vi "combined2.vi"() -> ()   [LabVIEW 2020]
uses:
  C:/Users/Public/Documents/Photometrics/PMQI-LabViewSamples/Examples/2018/Dependencies/PVCamNET.dll
  Dependencies/PVCamNET.dll
panel:
  out "SavingPath":string
  out "Saving":bool
  out "Capturing":bool
  in  "seq_save":bool
  in  "seq_start":bool
  in  "Path":path
  in  "FramesToCapture":u16
  in  "Full CCD Height":u16
  in  "Full CCD Width":u16
  in  "Full CCD":bool
  in  "Get ROI":bool
  in  "Height":u16
  in  "Y":u16
  in  "Width":u16
  in  "X":u16
  out "Trigger Mode":i32
  in  "Trigger In Behaviour":string(combo)
  out "Exp. out":i32
  in  "Trigger Out Behaviour":string(combo)
  out "Boolean":bool
  in  "Scan Direction Reset":bool
  out "Scan Line Time":dbl format="%#_14g"
  in  "Scan Width":dbl
  in  "Scan Line Delay":dbl
  in  "Scan Direction":string(combo)
  in  "Scan Mode":string(combo)
  in  "Exposure Time":dbl
  in  "Live":bool
  in  "Camera Status":bool
  in  "Uninit":bool
  in  "Live stop":bool
  in  "Live start":bool
  in  "Open":bool
  # "Description:\nThis code lets the user use programmable scan\n mode for live imaging.\n\nSteps to run:\n1. Click \"Run\"\n2. Click \"Open\"\n3. Enter Exposure Time\n4. Select Scan Mode. \n5. Set Scan Line Delay or Scan Width\n6. Select Scan Direction\n7. Click \"Live start\"\n8. Click \"Live stop\"\n9. Right click on CamWindow and add a ROI.\n10. Click \"Get ROI\"\n11. Click \"Live start\"\n12. Click \"Live stop\"\n13. Right click on CamWindow and delete a ROI.\n14. Click \"Close\""
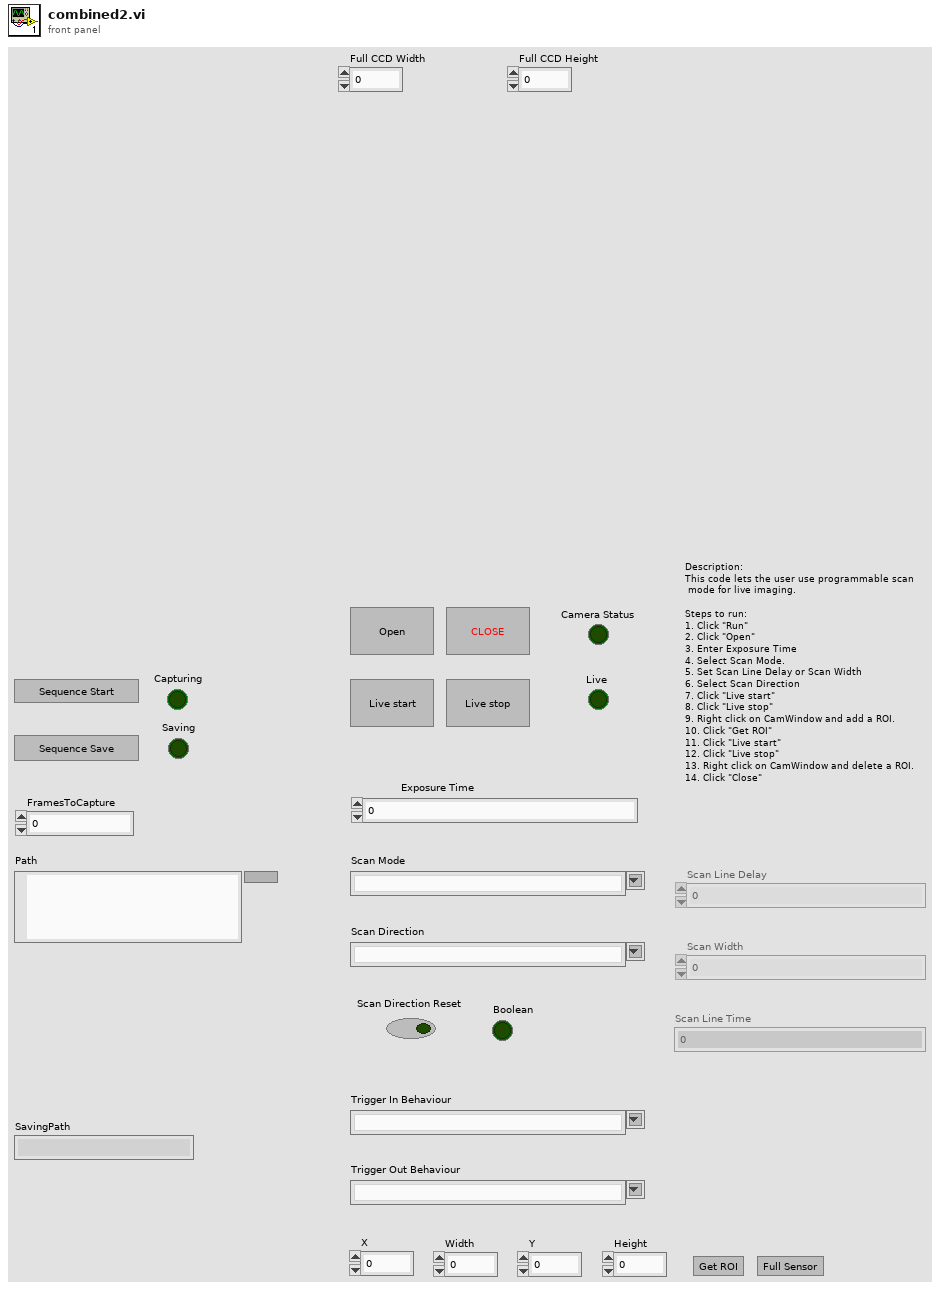
[diagram p1: front panel]
types:
  T1 = enum8{"Enabled", "Disabled", "Disabled and Grayed Out"}
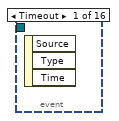
[diagram p2: hidden frame]
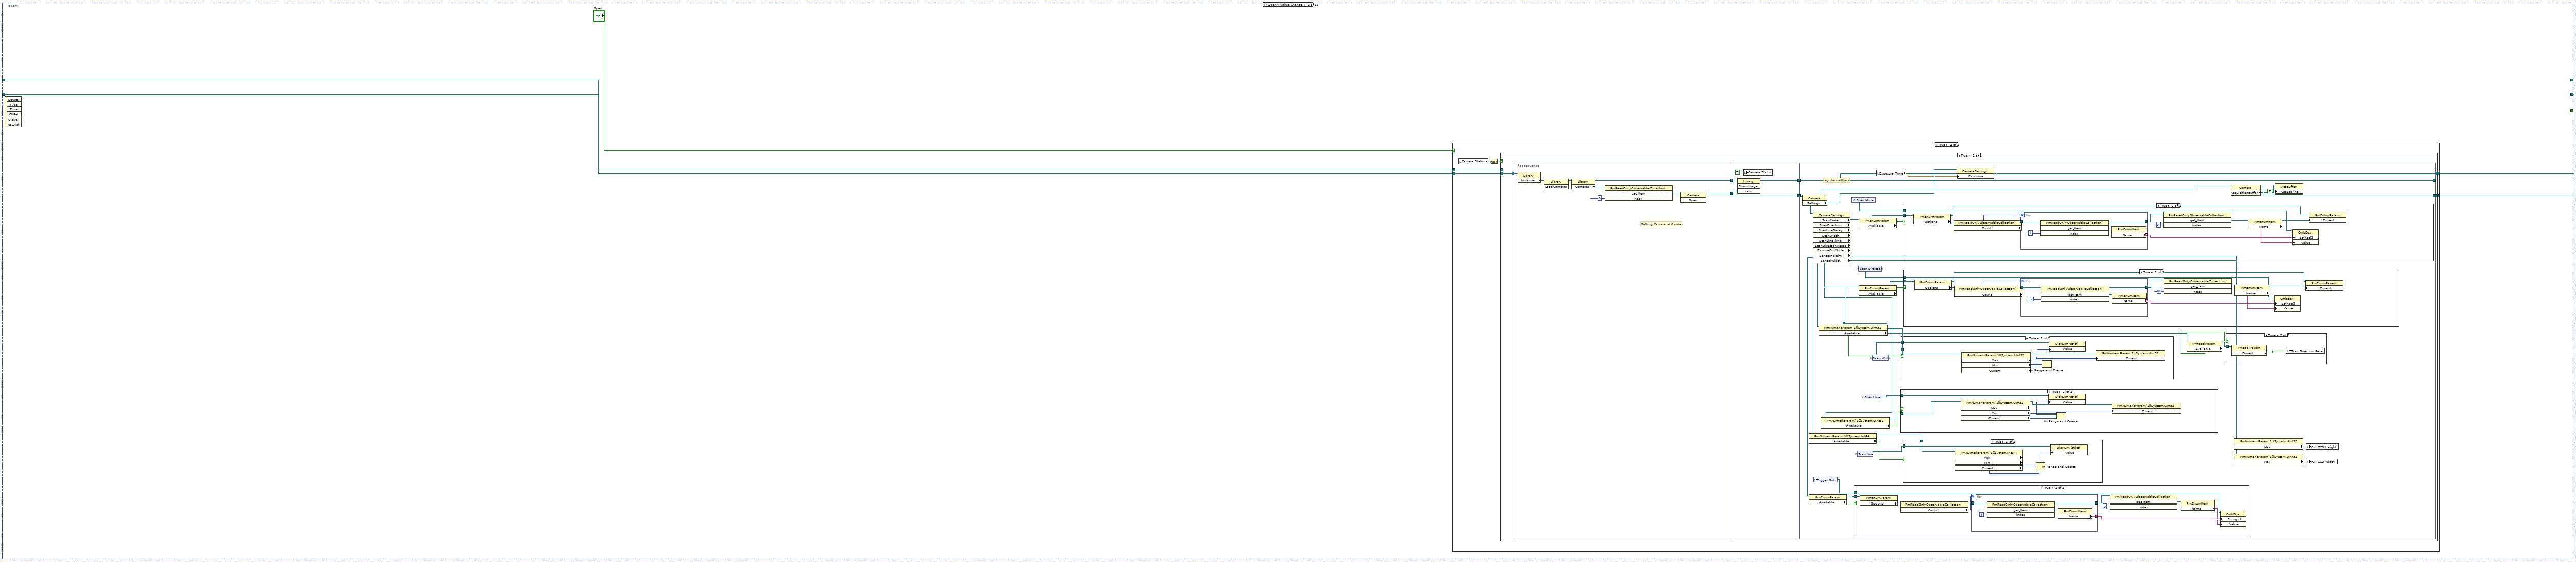
[diagram p3: hidden frame]
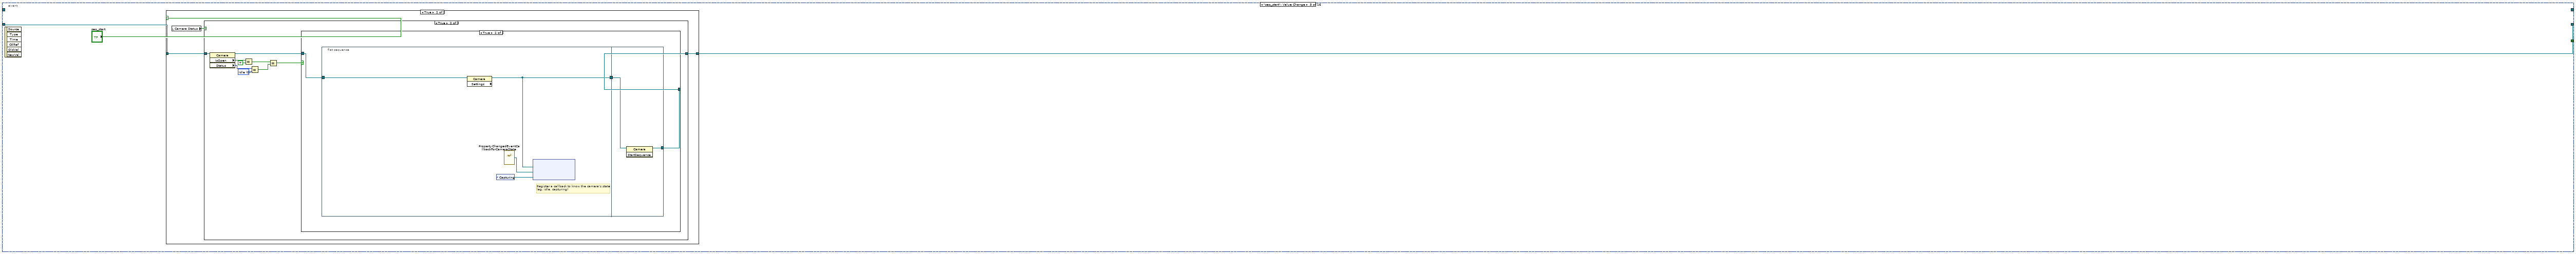
[diagram p13: hidden frame]
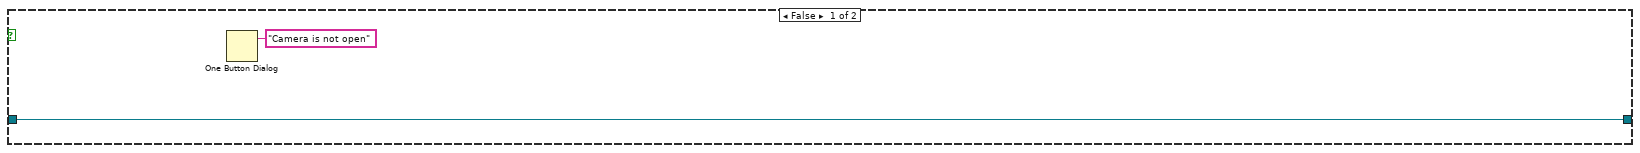
[diagram p15: hidden frame]
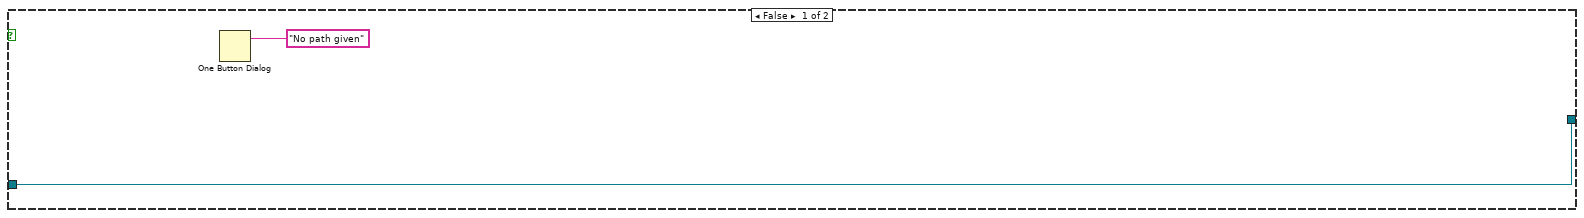
[diagram p18: hidden frame]
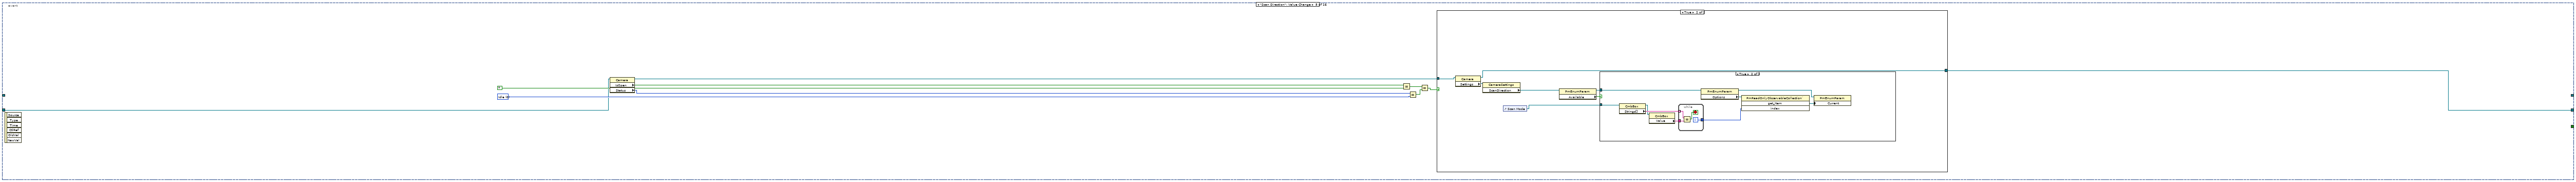
[diagram p20: hidden frame]
diagram:
  w15 = T1."Disabled and Grayed Out" ("Disabled")
  n1 = flat-sequence {
    tunnel: [w31] -> w30
    tunnel: w30 -> [w33]
    tunnel: [w32] -> w29
    tunnel: w29 -> [w859]
    frame #0 {
      n2 = property class="Library"() -> ("Instance"=w31:refnum<k24>)  [unwired: 2 in, 2 out]
    }
    frame #1 {
      n3 = while {
        tunnel: w33 -> [w38]
        shift-right: [w37] -> _
        shift-left: _ -> [w35]
        tunnel: [w36] -> w32
        stop <- w34 stop-if-true
        n4 = event shown="[3] \"seq_save\": Value Change" {
          selector: _ -> [_ _ _ _ _ _ _ _ _ _ _ _ _ _ _ _]
          dyn-events: _ -> [_ _ _ _ _ _ _ _ _ _ _ _ _ _ _ _]
          timeout: _ -> [_ _ _ _ _ _ _ _ _ _ _ _ _ _ _ _]
          tunnel: w38 -> [_ w43 _ _ _ _ _ _ w533 _ _ _ _ w776 _ w831]
          tunnel: [_ w42 w183 w214 w246 w278 w410 w474 w534 w601 w638 w711 w738 w777 w806 w832] -> w37
          tunnel: [_ w41 _ _ _ _ _ _ w533 _ _ _ _ w776 _ w831] -> w36
          tunnel: w35 -> [_ w40 w184 w213 w250 w279 w416 w476 w535 w602 w639 w712 w739 w778 w807 w833]
          tunnel: [_ _ _ _ _ _ _ _ _ _ _ _ _ _ _ w830] -> w34
          event Timeout {
            n5 = event-data() -> ()  [unwired: 1 in, 3 out]
          }
          event "Open": Value Change {
            n6 = event-data() -> ()  [unwired: 1 in, 6 out]
            n7 = case shown="True" "Open" {
              tunnel: w43 -> [w45 w51]
              tunnel: [w44 w50] -> w42
              tunnel: [w45 w49] -> w41
              tunnel: w40 -> [w44 w46]
              frame False {
              }
              frame True {
                n8 = local read "Camera Status"() -> (w48:bool)
                n9 = Not(x=w48) -> (.not. x?=w47:bool)
                n10 = case shown="True" w47 {
                  tunnel: w51 -> [w52 w58]
                  tunnel: [w53 w57] -> w50
                  tunnel: [w52 w56] -> w49
                  tunnel: w46 -> [w53 _]
                  frame False {
                  }
                  frame True {
                    n11 = flat-sequence {
                      tunnel: w58 -> [w63]
                      tunnel: [w65] -> w60
                      tunnel: [w64] -> w59
                      tunnel: w60 -> [w71]
                      tunnel: w59 -> [w72]
                      tunnel: [w72] -> w55
                      tunnel: [w70] -> w54
                      tunnel: [w111] -> w56
                      tunnel: [w91] -> w57
                      tunnel: w55 -> [w110]
                      tunnel: w54 -> [w111]
                      frame #0 {
                        # "Getting Camera at 0 index"
                        n12 = property class="Library"(reference=w63) -> ("Instance"=w62:refnum<k24>)  [unwired: 1 in, 2 out]
                        n13 = invoke class="Library" method="LoadCameras"(reference=w62) -> (reference out=w61:refnum<k24>)  [unwired: 2 in, 2 out]
                        n14 = property class="Library"(reference=w61) -> (reference out=w65:refnum<k24>, "Cameras"=w68:refnum<k24>)  [unwired: 1 in, 1 out]
                        n15 = invoke class="PmReadOnlyObservableCollection`" method="get_Item"(reference=w68, "index"=0) -> ("get_Item"=w66:refnum<k24>)  [unwired: 2 in, 3 out]
                        n16 = invoke class="Camera" method="Open"(reference=w66) -> (reference out=w64:refnum<k24>)  [unwired: 2 in, 2 out]
                      }
                      frame #1 {
                        n17 = invoke class="Library" method="ShowImage"(reference=w71, "cam"=w72) -> (reference out=w70:refnum<k24>)  [unwired: 2 in, 3 out]
                        n18 = local write "Camera Status"(TRUE ("Camera Status")) -> ()
                      }
                      frame #2 {
                        # "register callback"
                        n19 = property class="Camera"(reference=w110) -> (reference out=w92:refnum<k24>, "Settings"=w81:refnum<k24>)  [unwired: 1 in, 1 out]
                        n20 = property class="CameraSettings"(reference=w81) -> ("ScanMode"=w109:refnum<k24>, "ScanDirection"=w105:refnum<k24>, "ScanLineDelay"=w100:refnum<k24>, "ScanWidth"=w87:refnum<k24>, "ScanLineTime"=w79:refnum<k24>, "ScanDirectionReset"=w95:refnum<k24>, "ExposeOutMode"=w83:refnum<k24>, "SensorHeight"=w74:refnum<k24>, "SensorWidth"=w73:refnum<k24>)  [unwired: 1 in, 2 out]
                        n21 = property class="PmNumericParam`1[[System.Int64,"(reference=w79) -> (reference out=w77:refnum<k24>, "Available"=w78:bool)  [unwired: 1 in, 1 out]
                        n22 = property class="PmEnumParam"(reference=w83) -> (reference out=w84:refnum<k24>, "Available"=w85:bool)  [unwired: 1 in, 1 out]
                        n23 = control-ref of="Trigger Out Behaviour"() -> (w82:refnum<vi>)
                        n24 = property class="PmNumericParam`1[[System.UInt32"(reference=w100) -> (reference out=w98:refnum<k24>, "Available"=w99:bool)  [unwired: 1 in, 1 out]
                        n25 = property class="PmNumericParam`1[[System.UInt32"(reference=w87) -> (reference out=w86:refnum<k24>, "Available"=w88:bool)  [unwired: 1 in, 1 out]
                        n26 = control-ref of="Scan Mode"() -> (w106:refnum<vi>)
                        n27 = case shown="True" w85 {
                          tunnel: w84 -> [_ w121]
                          tunnel: w82 -> [_ w112]
                          frame False {
                          }
                          frame True {
                            n28 = property class="PmEnumParam"(reference=w121) -> ("Options"=w120:refnum<k24>)  [unwired: 1 in, 2 out]
                            n29 = property class="PmReadOnlyObservableCollection`"(reference=w120) -> (reference out=w118:refnum<k24>, "Count"=w119:i32)  [unwired: 1 in, 1 out]
                            n30 = for {
                              N: w119 -> [_]
                              tunnel: w118 -> [w126]
                              tunnel: [w123] -> w115
                              tunnel: [w122] -> w114 mode=indexing
                              i -> [w125]
                              n31 = invoke class="PmReadOnlyObservableCollection`" method="get_Item"(reference=w126, "index"=w125) -> (reference out=w123:refnum<k24>, "get_Item"=w124:refnum<k24>)  [unwired: 2 in, 2 out]
                              n32 = property class="PmEnumItem"(reference=w124) -> ("Name"=w122:string)  [unwired: 1 in, 2 out]
                            }
                            n33 = invoke class="PmReadOnlyObservableCollection`" method="get_Item"(reference=w115, "index"=0) -> ("get_Item"=w116:refnum<k24>)  [unwired: 2 in, 3 out]
                            n34 = property class="PmEnumItem"(reference=w116) -> ("Name"=w113:string)  [unwired: 1 in, 2 out]
                            n35 = property class="CmbBox"(reference=w112, "Strings[]"=w114, "Value"=w113) -> ()  [unwired: 1 in, 2 out]
                          }
                        }
                        n36 = control-ref of="Scan Line Time"() -> (w96:refnum<vi>)
                        n37 = control-ref of="Scan Direction"() -> (w102:refnum<vi>)
                        n38 = property class="PmEnumParam"(reference=w109) -> (reference out=w107:refnum<k24>, "Available"=w108:bool)  [unwired: 1 in, 1 out]
                        n39 = property class="PmEnumParam"(reference=w105) -> (reference out=w103:refnum<k24>, "Available"=w104:bool)  [unwired: 1 in, 1 out]
                        n40 = control-ref of="Scan Line Delay"() -> (w97:refnum<vi>)
                        n41 = control-ref of="Scan Width"() -> (w101:refnum<vi>)
                        n42 = local read "Exposure Time"() -> (w80:dbl)
                        n43 = case shown="True" w88 {
                          tunnel: w97 -> [_ w138]
                          tunnel: w86 -> [_ w137]
                          frame False {
                          }
                          frame True {
                            n44 = property class="PmNumericParam`1[[System.UInt32"(reference=w137) -> (reference out=w136:refnum<k24>, "Max"=w139:u32, "Min"=w140:u32, "Current"=w141:u32)  [unwired: 1 in, 1 out]
                            n45 = In Range and Coerce(upper limit=w139, x=w141, lower limit=w140) -> (coerced(x)=w135:u32)  [unwired: 1 out]
                            n46 = property class="DigNum (strict)"(reference=w138, "Value"=w135) -> ()  [unwired: 1 in, 2 out]
                            n47 = property class="PmNumericParam`1[[System.UInt32"(reference=w136, "Current"=w135) -> ()  [unwired: 1 in, 2 out]
                          }
                        }
                        n48 = case shown="True" w99 {
                          tunnel: w101 -> [_ w145]
                          tunnel: w98 -> [_ w144]
                          frame False {
                          }
                          frame True {
                            n49 = property class="PmNumericParam`1[[System.UInt32"(reference=w144) -> (reference out=w143:refnum<k24>, "Max"=w146:u32, "Min"=w147:u32, "Current"=w148:u32)  [unwired: 1 in, 1 out]
                            n50 = In Range and Coerce(upper limit=w146, x=w148, lower limit=w147) -> (coerced(x)=w142:u32)  [unwired: 1 out]
                            n51 = property class="DigNum (strict)"(reference=w145, "Value"=w142) -> ()  [unwired: 1 in, 2 out]
                            n52 = property class="PmNumericParam`1[[System.UInt32"(reference=w143, "Current"=w142) -> ()  [unwired: 1 in, 2 out]
                          }
                        }
                        n53 = case shown="True" w78 {
                          tunnel: w96 -> [_ w130]
                          tunnel: w77 -> [_ w129]
                          frame False {
                          }
                          frame True {
                            n54 = property class="PmNumericParam`1[[System.Int64,"(reference=w129) -> ("Max"=w131:i64, "Min"=w132:i64, "Current"=w133:i64)  [unwired: 1 in, 2 out]
                            n55 = In Range and Coerce(upper limit=w131, x=w133, lower limit=w132) -> (coerced(x)=w134:i64)  [unwired: 1 out]
                            n56 = property class="DigNum (strict)"(reference=w130, "Value"=w134) -> ()  [unwired: 1 in, 2 out]
                          }
                        }
                        n57 = case shown="True" w108 {
                          tunnel: w107 -> [_ w177]
                          tunnel: w106 -> [_ w169]
                          frame False {
                          }
                          frame True {
                            n58 = property class="PmEnumParam"(reference=w177) -> (reference out=w168:refnum<k24>, "Options"=w176:refnum<k24>)  [unwired: 1 in, 1 out]
                            n59 = property class="PmReadOnlyObservableCollection`"(reference=w176) -> (reference out=w174:refnum<k24>, "Count"=w175:i32)  [unwired: 1 in, 1 out]
                            n60 = for {
                              N: w175 -> [_]
                              tunnel: w174 -> [w182]
                              tunnel: [w179] -> w172
                              tunnel: [w178] -> w171 mode=indexing
                              i -> [w181]
                              n61 = invoke class="PmReadOnlyObservableCollection`" method="get_Item"(reference=w182, "index"=w181) -> (reference out=w179:refnum<k24>, "get_Item"=w180:refnum<k24>)  [unwired: 2 in, 2 out]
                              n62 = property class="PmEnumItem"(reference=w180) -> ("Name"=w178:string)  [unwired: 1 in, 2 out]
                            }
                            n63 = invoke class="PmReadOnlyObservableCollection`" method="get_Item"(reference=w172, "index"=0) -> ("get_Item"=w167:refnum<k24>)  [unwired: 2 in, 3 out]
                            n64 = property class="PmEnumItem"(reference=w167) -> (reference out=w166:refnum<k24>, "Name"=w170:string)  [unwired: 1 in, 1 out]
                            n65 = property class="CmbBox"(reference=w169, "Strings[]"=w171, "Value"=w170) -> ()  [unwired: 1 in, 2 out]
                            n66 = property class="PmEnumParam"(reference=w168, "Current"=w166) -> ()  [unwired: 1 in, 2 out]
                          }
                        }
                        n67 = case shown="True" w104 {
                          tunnel: w103 -> [_ w160]
                          tunnel: w102 -> [_ w151]
                          frame False {
                          }
                          frame True {
                            n68 = property class="PmEnumParam"(reference=w160) -> (reference out=w150:refnum<k24>, "Options"=w159:refnum<k24>)  [unwired: 1 in, 1 out]
                            n69 = property class="PmReadOnlyObservableCollection`"(reference=w159) -> (reference out=w157:refnum<k24>, "Count"=w158:i32)  [unwired: 1 in, 1 out]
                            n70 = for {
                              N: w158 -> [_]
                              tunnel: w157 -> [w165]
                              tunnel: [w162] -> w154
                              tunnel: [w161] -> w153 mode=indexing
                              i -> [w164]
                              n71 = invoke class="PmReadOnlyObservableCollection`" method="get_Item"(reference=w165, "index"=w164) -> (reference out=w162:refnum<k24>, "get_Item"=w163:refnum<k24>)  [unwired: 2 in, 2 out]
                              n72 = property class="PmEnumItem"(reference=w163) -> ("Name"=w161:string)  [unwired: 1 in, 2 out]
                            }
                            n73 = invoke class="PmReadOnlyObservableCollection`" method="get_Item"(reference=w154, "index"=0) -> ("get_Item"=w155:refnum<k24>)  [unwired: 2 in, 3 out]
                            n74 = property class="PmEnumItem"(reference=w155) -> (reference out=w149:refnum<k24>, "Name"=w152:string)  [unwired: 1 in, 1 out]
                            n75 = property class="CmbBox"(reference=w151, "Strings[]"=w153, "Value"=w152) -> ()  [unwired: 1 in, 2 out]
                            n76 = property class="PmEnumParam"(reference=w150, "Current"=w149) -> ()  [unwired: 1 in, 2 out]
                          }
                        }
                        n77 = property class="CameraSettings"(reference=w81, "Exposure"=w80) -> ()  [unwired: 1 in, 2 out]
                        n78 = property class="PmBoolParam"(reference=w95) -> (reference out=w93:refnum<k24>, "Available"=w94:bool)  [unwired: 1 in, 1 out]
                        n79 = case shown="True" w94 {
                          tunnel: w93 -> [_ w128]
                          frame False {
                          }
                          frame True {
                            n80 = property class="PmBoolParam"(reference=w128) -> ("Current"=w127:bool)  [unwired: 1 in, 2 out]
                            n81 = local write "Scan Direction Reset"(w127) -> ()
                          }
                        }
                        n82 = property class="Camera"(reference=w92) -> (reference out=w91:refnum<k24>, "AcquisitionBuffer"=w90:refnum<k24>)  [unwired: 1 in, 1 out]
                        n83 = property class="PmNumericParam`1[[System.UInt32"(reference=w74) -> ("Max"=w76:u32)  [unwired: 1 in, 2 out]
                        n84 = property class="PmNumericParam`1[[System.UInt32"(reference=w73) -> ("Max"=w75:u32)  [unwired: 1 in, 2 out]
                        n85 = property class="AcqBuffer"(reference=w90, "UseScaling"=TRUE) -> ()  [unwired: 1 in, 2 out]
                        n86 = local write "Full CCD Height"(w76) -> ()
                        n87 = local write "Full CCD Width"(w75) -> ()
                      }
                    }
                  }
                }
              }
            }
          }
          event "seq_start": Value Change {
            n88 = event-data() -> ()  [unwired: 1 in, 6 out]
            n89 = case shown="True" "seq_start" {
              tunnel: w184 -> [w186 w189]
              tunnel: [w186 w187] -> w183
              frame False {
              }
              frame True {
                n90 = local read "Camera Status"() -> (w188:bool)
                n91 = case shown="True" w188 {
                  tunnel: w189 -> [w190 w195]
                  tunnel: [w190 w192] -> w187
                  frame False {
                    n92 = One Button Dialog(message="Camera is not open") -> ()  [unwired: 1 in, 1 out]
                  }
                  frame True {
                    w200 = 0 items=["Idle", "Capturing"] ("Status")
                    n93 = property class="Camera"(reference=w195) -> (reference out=w194:refnum<k24>, "IsOpen"=w199:bool, "Status"=w201:i32)  [unwired: 1 in, 1 out]
                    n94 = Equal?(x=w199, y=TRUE) -> (x = y?=w197:bool)
                    n95 = Equal?(x=w201, y=w200) -> (x = y?=w196:bool)
                    n96 = Equal?(x=w197, y=w196) -> (x = y?=w193:bool)
                    n97 = case shown="True" w193 {
                      tunnel: w194 -> [w202 w205]
                      tunnel: [w202 w203] -> w192
                      frame False {
                      }
                      frame True {
                        n98 = flat-sequence {
                          tunnel: w205 -> [w207]
                          tunnel: [w206] -> w204
                          tunnel: w204 -> [w211]
                          tunnel: [w210] -> w203
                          frame #0 {
                            # "Register a callback to know the camera's state \n(eg. idle, capturing)"
                            n99 = property class="Camera" props=["Settings"](reference=w207) -> (reference out=w206:refnum<k24>)  [unwired: 1 in, 2 out]
                            n100 = control-ref of="Capturing"() -> (w208:refnum<vi>)
                            n101 = vi-ref "PropertyChangedEventCallbackForCameraState.vi"() -> ("vi reference"=w209:refnum<vi>)
                            n102 = node(w206, w209, w208) -> ()  [unwired: 2 in, 2 out]
                          }
                          frame #1 {
                            n103 = invoke class="Camera" method="StartSequence"(reference=w211) -> (reference out=w210:refnum<k24>)  [unwired: 2 in, 2 out]
                          }
                        }
                      }
                    }
                  }
                }
              }
            }
          }
          event "seq_save": Value Change {
            n104 = event-data() -> ()  [unwired: 1 in, 6 out]
            n105 = case shown="True" "seq_save" {
              tunnel: [w215 w223] -> w214
              tunnel: w213 -> [w215 w222]
              frame False {
              }
              frame True {
                n106 = local read "SavingPath"() -> (w219:string)
                n107 = Not Equal?(x=w219, y="\\") -> (x != y?=w217:bool)
                n108 = Not Equal?(x=w219, y="") -> (x != y?=w218:bool)
                n109 = And(x=w218, y=w217) -> (x .and. y?=w216:bool)
                n110 = case shown="True" w216 {
                  tunnel: [w224 w227] -> w223
                  tunnel: w222 -> [w224 w226]
                  frame False {
                    n111 = One Button Dialog(message="No path given") -> ()  [unwired: 1 in, 1 out]
                  }
                  frame True {
                    w234 = 0 items=["Idle", "Capturing"] ("Status")
                    n112 = property class="Camera"(reference=w226) -> (reference out=w229:refnum<k24>, "IsOpen"=w233:bool, "Status"=w235:i32)  [unwired: 1 in, 1 out]
                    n113 = Equal?(x=w233, y=TRUE) -> (x = y?=w231:bool)
                    n114 = Equal?(x=w235, y=w234) -> (x = y?=w230:bool)
                    n115 = Equal?(x=w231, y=w230) -> (x = y?=w228:bool)
                    n116 = case shown="True" w228 {
                      tunnel: w229 -> [w236 w239]
                      tunnel: [w236 w238] -> w227
                      frame False {
                      }
                      frame True {
                        n117 = flat-sequence {
                          tunnel: [w241] -> w237
                          tunnel: w239 -> [w240]
                          tunnel: [w244] -> w238
                          tunnel: w237 -> [w244]
                          frame #0 {
                            # "Save all the frames in the buffer to a Tiff image"
                            n118 = property class="Camera"(reference=w240) -> (reference out=w241:refnum<k24>, "AcquisitionBuffer"=w243:refnum<k24>)  [unwired: 1 in, 1 out]
                            n119 = local write "Saving"(TRUE ("Camera Status")) -> ()
                            n120 = invoke class="AcqBuffer" method="SaveAsTiff"(reference=w243) -> ()  [unwired: 2 in, 3 out]
                          }
                          frame #1 {
                            n121 = local write "Saving"(FALSE ("Camera Status")) -> ()
                          }
                        }
                      }
                    }
                  }
                }
              }
            }
          }
          event "Scan Direction": Value Change {
            w254 = 0 items=["Idle", "Capturing"] ("Status")
            n122 = event-data() -> ()  [unwired: 1 in, 6 out]
            n123 = property class="Camera"(reference=w250) -> (reference out=w247:refnum<k24>, "IsOpen"=w253:bool, "Status"=w255:i32)  [unwired: 1 in, 1 out]
            n124 = Equal?(x=w253, y=TRUE) -> (x = y?=w249:bool)
            n125 = Equal?(x=w255, y=w254) -> (x = y?=w251:bool)
            n126 = Equal?(x=w249, y=w251) -> (x = y?=w248:bool)
            n127 = case shown="True" w248 {
              tunnel: w247 -> [w256 w260]
              tunnel: [w256 w257] -> w246
              frame False {
              }
              frame True {
                n128 = property class="Camera"(reference=w260) -> (reference out=w257:refnum<k24>, "Settings"=w261:refnum<k24>)  [unwired: 1 in, 1 out]
                n129 = property class="CameraSettings"(reference=w261) -> ("ScanDirection"=w259:refnum<k24>)  [unwired: 1 in, 2 out]
                n130 = control-ref of="Scan Mode"() -> (w258:refnum<vi>)
                n131 = property class="PmEnumParam"(reference=w259) -> (reference out=w262:refnum<k24>, "Available"=w263:bool)  [unwired: 1 in, 1 out]
                n132 = case shown="True" w263 {
                  tunnel: w262 -> [_ w271]
                  tunnel: w258 -> [_ w264]
                  frame False {
                  }
                  frame True {
                    n133 = property class="CmbBox"(reference=w264) -> (reference out=w266:refnum<vi>, "Strings[]"=w272:string[])  [unwired: 1 in, 1 out]
                    n134 = property class="CmbBox"(reference=w266) -> ("Value"=w265:string)  [unwired: 1 in, 2 out]
                    n135 = while {
                      tunnel: w272 -> [w276] mode=indexing
                      tunnel: [w274] -> w269
                      tunnel: w265 -> [w273]
                      i -> [w274]
                      stop <- w275 stop-if-true
                      n136 = Equal?(x=w276, y=w273) -> (x = y?=w275:bool)
                    }
                    n137 = property class="PmEnumParam"(reference=w271) -> (reference out=w268:refnum<k24>, "Options"=w270:refnum<k24>)  [unwired: 1 in, 1 out]
                    n138 = invoke class="PmReadOnlyObservableCollection`" method="get_Item"(reference=w270, "index"=w269) -> ("get_Item"=w267:refnum<k24>)  [unwired: 2 in, 3 out]
                    n139 = property class="PmEnumParam"(reference=w268, "Current"=w267) -> ()  [unwired: 1 in, 2 out]
                  }
                }
              }
            }
          }
          event "Scan Mode", "Scan Direction Reset": Value Change {
            n140 = event-data() -> ()  [unwired: 1 in, 6 out]
            n141 = local read "Camera Status"() -> (w277:bool)
            n142 = case shown="True" w277 {
              tunnel: w279 -> [w280 w285]
              tunnel: [w280 w283] -> w278
              frame False {
                n143 = One Button Dialog(message="Camera is not open") -> ()  [unwired: 1 in, 1 out]
              }
              frame True {
                w290 = 0 items=["Idle", "Capturing"] ("Status")
                n144 = property class="Camera"(reference=w285) -> (reference out=w284:refnum<k24>, "IsOpen"=w289:bool, "Status"=w291:i32)  [unwired: 1 in, 1 out]
                n145 = Equal?(x=w289, y=TRUE) -> (x = y?=w287:bool)
                n146 = Equal?(x=w291, y=w290) -> (x = y?=w286:bool)
                n147 = Equal?(x=w287, y=w286) -> (x = y?=w282:bool)
                n148 = case shown="True" w282 {
                  tunnel: w284 -> [w292 w331]
                  tunnel: [w292 w326] -> w283
                  frame False {
                  }
                  frame True {
                    # "For Scan mode type if Auto is chosen then Scan Width and Scan Line Delay are not configurable.\nIf Line Delay is chosen then Scan Line is configurable, but Scan Width is not configurable.\nSimilarly if Scan Delay is chosen then Scan Line Delay is configurable, but Scan Width is not configurable."
                    n149 = property class="Camera"(reference=w331) -> (reference out=w326:refnum<k24>, "Settings"=w330:refnum<k24>)  [unwired: 1 in, 1 out]
                    n150 = property class="CameraSettings"(reference=w330) -> (error out=w323:errorcluster, "ScanMode"=w329:refnum<k24>, "ScanDirection"=w325:refnum<k24>, "ScanWidth"=w321:refnum<k24>, "ScanLineDelay"=w320:refnum<k24>, "ScanLineTime"=w309:refnum<k24>, "ScanDirectionReset"=w298:refnum<k24>)  [unwired: 1 in, 1 out]
                    n151 = control-ref of="Scan Line Delay"() -> (w300:refnum<vi>)
                    n152 = control-ref of="Scan Line Time"() -> (w303:refnum<vi>)
                    n153 = control-ref of="Scan Width"() -> (w316:refnum<vi>)
                    n154 = property class="PmEnumParam"(reference=w329, error in=w323) -> (reference out=w327:refnum<k24>, error out=w324:errorcluster, "Available"=w328:bool)
                    n155 = control-ref of="Scan Mode"() -> (w322:refnum<vi>)
                    n156 = control-ref of="Scan Direction"() -> (w319:refnum<vi>)
                    n157 = case shown="True" w328 {
                      tunnel: w327 -> [_ w404]
                      tunnel: w322 -> [_ w399]
                      tunnel: w324 -> [w392 w398]
                      tunnel: [w392 w393] -> w308
                      frame False {
                      }
                      frame True {
                        n158 = property class="CmbBox"(reference=w399) -> (reference out=w400:refnum<vi>, "Strings[]"=w405:string[])  [unwired: 1 in, 1 out]
                        n159 = property class="CmbBox"(reference=w400) -> ("Value"=w395:string)  [unwired: 1 in, 2 out]
                        n160 = while {
                          tunnel: w405 -> [w409] mode=indexing
                          tunnel: [w407] -> w402
                          tunnel: w395 -> [w406]
                          i -> [w407]
                          stop <- w408 stop-if-true
                          n161 = Equal?(x=w409, y=w406) -> (x = y?=w408:bool)
                        }
                        n162 = property class="PmEnumParam"(reference=w404, error in=w398) -> (reference out=w401:refnum<k24>, error out=w397:errorcluster, "Options"=w403:refnum<k24>)
                        n163 = invoke class="PmReadOnlyObservableCollection`" method="get_Item"(reference=w403, error in=w397, "index"=w402) -> (error out=w396:errorcluster, "get_Item"=w394:refnum<k24>)  [unwired: 1 in, 2 out]
                        n164 = property class="PmEnumParam" props=["Current", "IsReadOnly"](reference=w401, error in=w396, "Current"=w394) -> (error out=w393:errorcluster)  [unwired: 2 out]
                      }
                    }
                    n165 = property class="PmEnumParam"(reference=w325, error in=w308) -> (reference out=w317:refnum<k24>, error out=w311:errorcluster, "Available"=w318:bool)
                    n166 = case shown="True" w318 {
                      tunnel: w317 -> [_ w386]
                      tunnel: w319 -> [_ w378]
                      tunnel: w311 -> [w370 w377]
                      tunnel: [w370 w371] -> w310
                      frame False {
                      }
                      frame True {
                        n167 = property class="PmEnumParam"(reference=w386, error in=w377) -> (reference out=w372:refnum<k24>, error out=w376:errorcluster, "Options"=w385:refnum<k24>)
                        n168 = property class="PmReadOnlyObservableCollection`"(reference=w385) -> (reference out=w383:refnum<k24>, "Count"=w384:i32)  [unwired: 1 in, 1 out]
                        n169 = for {
                          N: w384 -> [_]
                          tunnel: w383 -> [w391]
                          tunnel: [w388] -> w381
                          tunnel: [w387] -> w380 mode=indexing
                          i -> [w390]
                          n170 = invoke class="PmReadOnlyObservableCollection`" method="get_Item"(reference=w391, "index"=w390) -> (reference out=w388:refnum<k24>, "get_Item"=w389:refnum<k24>)  [unwired: 2 in, 2 out]
                          n171 = property class="PmEnumItem"(reference=w389) -> ("Name"=w387:string)  [unwired: 1 in, 2 out]
                        }
                        n172 = invoke class="PmReadOnlyObservableCollection`" method="get_Item"(reference=w381, error in=w376, "index"=0) -> (error out=w375:errorcluster, "get_Item"=w373:refnum<k24>)  [unwired: 1 in, 2 out]
                        n173 = property class="PmEnumItem"(reference=w373, error in=w375) -> (error out=w374:errorcluster, "Name"=w379:string)  [unwired: 1 out]
                        n174 = property class="CmbBox"(reference=w378, error in=w374, "Strings[]"=w380, "Value"=w379) -> (error out=w371:errorcluster)  [unwired: 1 out]
                        n175 = property class="PmEnumParam"(reference=w372, "Current"=w373) -> ()  [unwired: 1 in, 2 out]
                      }
                    }
                    n176 = property class="PmNumericParam`1[[System.UInt32"(reference=w321, error in=w310) -> (reference out=w314:refnum<k24>, error out=w313:errorcluster, "Available"=w315:bool)
                    n177 = case shown="True" w315 {
                      tunnel: w316 -> [_ w366]
                      tunnel: w314 -> [_ w363]
                      tunnel: w313 -> [w360 w365]
                      tunnel: [w360 w364] -> w312
                      frame False {
                      }
                      frame True {
                        n178 = property class="PmNumericParam`1[[System.UInt32"(reference=w363) -> ("Current"=w367:u32, "IsReadOnly"=w362:bool)  [unwired: 1 in, 2 out]
                        n179 = case shown="False" w362 {
                          tunnel: [T1."Enabled" ("Disabled") T1."Disabled and Grayed Out" ("Disabled")] -> w361
                          frame False {
                          }
                          frame True {
                          }
                        }
                        n180 = property class="DigNum (strict)"(reference=w366, error in=w365, "Value"=w367, "DisabledEnum"=w361) -> (error out=w364:errorcluster)  [unwired: 1 out]
                      }
                    }
                    n181 = property class="PmNumericParam`1[[System.UInt32"(reference=w320, error in=w312) -> (reference out=w305:refnum<k24>, error out=w299:errorcluster, "Available"=w306:bool)
                    n182 = case shown="True" w306 {
                      tunnel: w300 -> [_ w356]
                      tunnel: w305 -> [_ w353]
                      tunnel: w299 -> [w350 w355]
                      tunnel: [w350 w354] -> w302
                      frame False {
                      }
                      frame True {
                        n183 = property class="PmNumericParam`1[[System.UInt32"(reference=w353) -> ("Current"=w357:u32, "IsReadOnly"=w352:bool)  [unwired: 1 in, 2 out]
                        n184 = case shown="False" w352 {
                          tunnel: [T1."Enabled" ("Disabled") T1."Disabled and Grayed Out" ("Disabled")] -> w351
                          frame False {
                          }
                          frame True {
                          }
                        }
                        n185 = property class="DigNum (strict)"(reference=w356, error in=w355, "Value"=w357, "DisabledEnum"=w351) -> (error out=w354:errorcluster)  [unwired: 1 out]
                      }
                    }
                    n186 = property class="PmNumericParam`1[[System.Int64,"(reference=w309, error in=w302) -> (reference out=w304:refnum<k24>, error out=w301:errorcluster, "Available"=w307:bool)
                    n187 = case shown="True" w307 {
                      tunnel: w303 -> [_ w346]
                      tunnel: w304 -> [_ w343]
                      tunnel: w301 -> [w340 w345]
                      tunnel: [w340 w344] -> w294
                      frame False {
                      }
                      frame True {
                        n188 = property class="PmNumericParam`1[[System.Int64,"(reference=w343) -> ("Current"=w347:i64, "IsReadOnly"=w342:bool)  [unwired: 1 in, 2 out]
                        n189 = case shown="False" w342 {
                          tunnel: [T1."Enabled" ("Disabled") T1."Disabled and Grayed Out" ("Disabled")] -> w341
                          frame False {
                          }
                          frame True {
                          }
                        }
                        n190 = property class="DigNum (strict)"(reference=w346, error in=w345, "Value"=w347, "DisabledEnum"=w341) -> (error out=w344:errorcluster)  [unwired: 1 out]
                      }
                    }
                    n191 = property class="PmBoolParam"(reference=w298, error in=w294) -> (reference out=w296:refnum<k24>, error out=w293:errorcluster, "Available"=w297:bool)
                    n192 = control-ref of="Scan Direction Reset"() -> (w295:refnum<vi>)
                    n193 = case shown="True" w297 {
                      tunnel: w296 -> [_ w337]
                      tunnel: w295 -> [_ w339]
                      tunnel: w293 -> [_ w334]
                      frame False {
                      }
                      frame True {
                        n194 = property class="Bool (strict)"(reference=w339, error in=w334) -> (error out=w333:errorcluster, "Value"=w338:bool)  [unwired: 1 out]
                        n195 = property class="PmBoolParam"(reference=w337, error in=w333, "Current"=w338) -> (reference out=w336:refnum<k24>, error out=w332:errorcluster)
                        n196 = property class="PmBoolParam"(reference=w336, error in=w332) -> ("Current"=w335:bool)  [unwired: 2 out]
                        n197 = local write "Boolean"(w335) -> ()
                      }
                    }
                  }
                }
              }
            }
          }
          event "Scan Line Delay": Value Change {
            w421 = 0 items=["Idle", "Capturing"] ("Status")
            n198 = event-data() -> ()  [unwired: 1 in, 6 out]
            n199 = property class="Camera"(reference=w416) -> (reference out=w415:refnum<k24>, "IsOpen"=w420:bool, "Status"=w422:i32)  [unwired: 1 in, 1 out]
            n200 = Equal?(x=w420, y=TRUE) -> (x = y?=w418:bool)
            n201 = Equal?(x=w422, y=w421) -> (x = y?=w417:bool)
            n202 = Equal?(x=w418, y=w417) -> (x = y?=w414:bool)
            n203 = control-ref of="Scan Line Time"() -> (w411:refnum<vi>)
            n204 = control-ref of="Scan Line Delay"() -> (w412:refnum<vi>)
            n205 = control-ref of="Scan Width"() -> (w413:refnum<vi>)
            n206 = case shown="True" w414 {
              tunnel: w415 -> [w423 w445]
              tunnel: [w423 w444] -> w410
              tunnel: w412 -> [_ w443]
              tunnel: w413 -> [_ w442]
              tunnel: w411 -> [_ w426]
              frame False {
              }
              frame True {
                n207 = property class="Camera"(reference=w445) -> (reference out=w444:refnum<k24>, "Settings"=w441:refnum<k24>)  [unwired: 1 in, 1 out]
                n208 = property class="CameraSettings"(reference=w441) -> (reference out=w431:refnum<k24>, error out=w437:errorcluster, "ScanLineDelay"=w440:refnum<k24>)  [unwired: 1 in]
                n209 = property class="PmNumericParam`1[[System.UInt32"(reference=w440, error in=w437) -> (reference out=w438:refnum<k24>, error out=w436:errorcluster, "Available"=w439:bool)
                n210 = case shown="True" w439 {
                  tunnel: w443 -> [_ w462]
                  tunnel: w438 -> [_ w461]
                  tunnel: w436 -> [w457 w460]
                  tunnel: [w457 w458] -> w432
                  frame False {
                  }
                  frame True {
                    n211 = property class="PmNumericParam`1[[System.UInt32"(reference=w461) -> (reference out=w465:refnum<k24>, "Max"=w463:u32, "Min"=w464:u32)  [unwired: 1 in, 1 out]
                    n212 = property class="DigNum (strict)"(reference=w462, error in=w460) -> (reference out=w469:refnum<vi>, error out=w459:errorcluster, "Value"=w468:dbl)
                    n213 = In Range and Coerce(upper limit=w463, x=w468, lower limit=w464) -> (coerced(x)=w467:dbl)  [unwired: 1 out]
                    n214 = property class="PmNumericParam`1[[System.UInt32"(reference=w465, "Current"=w467) -> (reference out=w466:refnum<k24>)  [unwired: 1 in, 1 out]
                    n215 = property class="PmNumericParam`1[[System.UInt32"(reference=w466) -> ("Current"=w470:u32)  [unwired: 1 in, 2 out]
                    n216 = property class="DigNum (strict)"(reference=w469, error in=w459, "Value"=w470) -> (error out=w458:errorcluster)  [unwired: 1 out]
                  }
                }
                n217 = property class="CameraSettings"(reference=w431) -> ("ScanWidth"=w430:refnum<k24>, "ScanLineTime"=w429:refnum<k24>)  [unwired: 1 in, 2 out]
                n218 = property class="PmNumericParam`1[[System.UInt32"(reference=w430, error in=w432) -> (reference out=w434:refnum<k24>, error out=w433:errorcluster, "Available"=w435:bool)
                n219 = case shown="True" w435 {
                  tunnel: w442 -> [_ w453]
                  tunnel: w434 -> [_ w456]
                  tunnel: w433 -> [w451 w454]
                  tunnel: [w451 w455] -> w425
                  frame False {
                  }
                  frame True {
                    n220 = property class="PmNumericParam`1[[System.UInt32"(reference=w456) -> ("Current"=w452:u32)  [unwired: 1 in, 2 out]
                    n221 = property class="DigNum (strict)"(reference=w453, error in=w454, "Value"=w452) -> (error out=w455:errorcluster)  [unwired: 1 out]
                  }
                }
                n222 = property class="PmNumericParam`1[[System.Int64,"(reference=w429, error in=w425) -> (reference out=w427:refnum<k24>, error out=w424:errorcluster, "Available"=w428:bool)
                n223 = case shown="True" w428 {
                  tunnel: w427 -> [_ w450]
                  tunnel: w426 -> [_ w448]
                  tunnel: w424 -> [_ w447]
                  frame False {
                  }
                  frame True {
                    n224 = property class="PmNumericParam`1[[System.Int64,"(reference=w450, error in=w447) -> (error out=w446:errorcluster, "Current"=w449:i64)  [unwired: 1 out]
                    n225 = property class="DigNum (strict)"(reference=w448, error in=w446, "Value"=w449) -> ()  [unwired: 2 out]
                  }
                }
              }
            }
          }
          event "Scan Width": Value Change {
            w482 = 0 items=["Idle", "Capturing"] ("Status")
            n226 = event-data() -> ()  [unwired: 1 in, 6 out]
            n227 = property class="Camera"(reference=w476) -> (reference out=w475:refnum<k24>, "IsOpen"=w481:bool, "Status"=w483:i32)  [unwired: 1 in, 1 out]
            n228 = Equal?(x=w481, y=TRUE) -> (x = y?=w479:bool)
            n229 = Equal?(x=w483, y=w482) -> (x = y?=w478:bool)
            n230 = Equal?(x=w479, y=w478) -> (x = y?=w477:bool)
            n231 = control-ref of="Scan Line Time"() -> (w471:refnum<vi>)
            n232 = control-ref of="Scan Width"() -> (w473:refnum<vi>)
            n233 = control-ref of="Scan Line Delay"() -> (w472:refnum<vi>)
            n234 = case shown="True" w477 {
              tunnel: w475 -> [w484 w506]
              tunnel: [w484 w505] -> w474
              tunnel: w473 -> [_ w504]
              tunnel: w472 -> [_ w503]
              tunnel: w471 -> [_ w488]
              frame False {
              }
              frame True {
                n235 = property class="Camera"(reference=w506) -> (reference out=w505:refnum<k24>, "Settings"=w502:refnum<k24>)  [unwired: 1 in, 1 out]
                n236 = property class="CameraSettings"(reference=w502) -> (reference out=w485:refnum<k24>, error out=w498:errorcluster, "ScanWidth"=w501:refnum<k24>)  [unwired: 1 in]
                n237 = property class="PmNumericParam`1[[System.UInt32"(reference=w501, error in=w498) -> (reference out=w499:refnum<k24>, error out=w497:errorcluster, "Available"=w500:bool)
                n238 = case shown="True" w500 {
                  tunnel: w504 -> [_ w523]
                  tunnel: w499 -> [_ w522]
                  tunnel: w497 -> [w518 w521]
                  tunnel: [w518 w519] -> w493
                  frame False {
                  }
                  frame True {
                    n239 = property class="PmNumericParam`1[[System.UInt32"(reference=w522) -> (reference out=w526:refnum<k24>, "Max"=w524:u32, "Min"=w525:u32)  [unwired: 1 in, 1 out]
                    n240 = property class="DigNum (strict)"(reference=w523, error in=w521) -> (reference out=w530:refnum<vi>, error out=w520:errorcluster, "Value"=w529:dbl)
                    n241 = In Range and Coerce(upper limit=w524, x=w529, lower limit=w525) -> (coerced(x)=w528:dbl)  [unwired: 1 out]
                    n242 = property class="PmNumericParam`1[[System.UInt32"(reference=w526, "Current"=w528) -> (reference out=w527:refnum<k24>)  [unwired: 1 in, 1 out]
                    n243 = property class="PmNumericParam`1[[System.UInt32"(reference=w527) -> ("Current"=w531:u32)  [unwired: 1 in, 2 out]
                    n244 = property class="DigNum (strict)"(reference=w530, error in=w520, "Value"=w531) -> (error out=w519:errorcluster)  [unwired: 1 out]
                  }
                }
                n245 = property class="CameraSettings"(reference=w485) -> ("ScanLineDelay"=w492:refnum<k24>, "ScanLineTime"=w491:refnum<k24>)  [unwired: 1 in, 2 out]
                n246 = property class="PmNumericParam`1[[System.UInt32"(reference=w492, error in=w493) -> (reference out=w495:refnum<k24>, error out=w494:errorcluster, "Available"=w496:bool)
                n247 = case shown="True" w496 {
                  tunnel: w503 -> [_ w514]
                  tunnel: w495 -> [_ w517]
                  tunnel: w494 -> [w512 w515]
                  tunnel: [w512 w516] -> w487
                  frame False {
                  }
                  frame True {
                    n248 = property class="PmNumericParam`1[[System.UInt32"(reference=w517) -> ("Current"=w513:u32)  [unwired: 1 in, 2 out]
                    n249 = property class="DigNum (strict)"(reference=w514, error in=w515, "Value"=w513) -> (error out=w516:errorcluster)  [unwired: 1 out]
                  }
                }
                n250 = property class="PmNumericParam`1[[System.Int64,"(reference=w491, error in=w487) -> (reference out=w489:refnum<k24>, error out=w486:errorcluster, "Available"=w490:bool)
                n251 = case shown="True" w490 {
                  tunnel: w489 -> [_ w511]
                  tunnel: w488 -> [_ w509]
                  tunnel: w486 -> [_ w508]
                  frame False {
                  }
                  frame True {
                    n252 = property class="PmNumericParam`1[[System.Int64,"(reference=w511, error in=w508) -> (error out=w507:errorcluster, "Current"=w510:i64)  [unwired: 1 out]
                    n253 = property class="DigNum (strict)"(reference=w509, error in=w507, "Value"=w510) -> ()  [unwired: 2 out]
                  }
                }
              }
            }
          }
          event "Trigger In Behaviour", "Trigger Out Behaviour": Value Change {
            n254 = event-data() -> ()  [unwired: 1 in, 6 out]
            n255 = local read "Camera Status"() -> (w532:bool)
            n256 = case shown="True" w532 {
              tunnel: w535 -> [w537 w541]
              tunnel: [w537 w538] -> w534
              frame False {
                n257 = One Button Dialog(message="Camera is not open") -> ()  [unwired: 1 in, 1 out]
              }
              frame True {
                w546 = 0 items=["Idle", "Capturing"] ("Status")
                n258 = property class="Camera"(reference=w541) -> (reference out=w539:refnum<k24>, "IsOpen"=w545:bool, "Status"=w547:i32)  [unwired: 1 in, 1 out]
                n259 = Equal?(x=w545, y=TRUE) -> (x = y?=w543:bool)
                n260 = Equal?(x=w547, y=w546) -> (x = y?=w542:bool)
                n261 = Equal?(x=w543, y=w542) -> (x = y?=w540:bool)
                n262 = case shown="True" w540 {
                  tunnel: w539 -> [w548 w570]
                  tunnel: [w548 w562] -> w538
                  frame False {
                  }
                  frame True {
                    n263 = property class="Camera"(reference=w570) -> (reference out=w562:refnum<k24>, "Settings"=w557:refnum<k24>)  [unwired: 1 in, 1 out]
                    n264 = control-ref of="Trigger In Behaviour"() -> (w552:refnum<vi>)
                    n265 = control-ref of="Trigger Mode"() -> (w553:refnum<vi>)
                    n266 = control-ref of="Trigger Out Behaviour"() -> (w558:refnum<vi>)
                    n267 = control-ref of="Exp. out"() -> (w559:refnum<vi>)
                    n268 = property class="CameraSettings"(reference=w557) -> (reference out=w556:refnum<k24>, "ExposureTime"=w555:refnum<k24>, "ExposureMode"=w549:refnum<k24>, "ExposeOutMode"=w554:refnum<k24>)  [unwired: 1 in, 1 out]
                    n269 = property class="PmEnumParam"(reference=w554) -> (reference out=w560:refnum<k24>, "Available"=w561:bool)  [unwired: 1 in, 1 out]
                    n270 = property class="PmEnumParam"(reference=w549) -> (reference out=w551:refnum<k24>, "Available"=w550:bool)  [unwired: 1 in, 1 out]
                    n271 = property class="PmNumericParam`1[[System.UInt64"(reference=w555) -> (reference out=w567:refnum<k24>, "Max"=w569:u64, "Min"=w568:u64)  [unwired: 1 in, 1 out]
                    n272 = case shown="True" w561 {
                      tunnel: w560 -> [_ w595]
                      tunnel: w559 -> [_ w589]
                      tunnel: w558 -> [_ w586]
                      frame False {
                      }
                      frame True {
                        n273 = property class="CmbBox"(reference=w586) -> (reference out=w588:refnum<vi>, "Strings[]"=w596:string[])  [unwired: 1 in, 1 out]
                        n274 = property class="CmbBox"(reference=w588) -> ("Value"=w587:string)  [unwired: 1 in, 2 out]
                        n275 = while {
                          tunnel: w596 -> [w600] mode=indexing
                          tunnel: [w598] -> w593
                          tunnel: w587 -> [w597]
                          i -> [w598]
                          stop <- w599 stop-if-true
                          n276 = Equal?(x=w600, y=w597) -> (x = y?=w599:bool)
                        }
                        n277 = property class="PmEnumParam"(reference=w595) -> (reference out=w592:refnum<k24>, "Options"=w594:refnum<k24>)  [unwired: 1 in, 1 out]
                        n278 = invoke class="PmReadOnlyObservableCollection`" method="get_Item"(reference=w594, "index"=w593) -> ("get_Item"=w591:refnum<k24>)  [unwired: 2 in, 3 out]
                        n279 = property class="PmEnumItem"(reference=w591) -> ("Value"=w590:i32)  [unwired: 1 in, 2 out]
                        n280 = property class="PmEnumParam"(reference=w592, "Current"=w591) -> ()  [unwired: 1 in, 2 out]
                        n281 = property class="DigNum (strict)"(reference=w589, "Value"=w590) -> ()  [unwired: 1 in, 2 out]
                      }
                    }
                    n282 = case shown="True" w550 {
                      tunnel: w551 -> [_ w580]
                      tunnel: w553 -> [_ w574]
                      tunnel: w552 -> [_ w571]
                      frame False {
                      }
                      frame True {
                        n283 = property class="CmbBox"(reference=w571) -> (reference out=w573:refnum<vi>, "Strings[]"=w581:string[])  [unwired: 1 in, 1 out]
                        n284 = property class="CmbBox"(reference=w573) -> ("Value"=w572:string)  [unwired: 1 in, 2 out]
                        n285 = while {
                          tunnel: w581 -> [w585] mode=indexing
                          tunnel: [w583] -> w578
                          tunnel: w572 -> [w582]
                          i -> [w583]
                          stop <- w584 stop-if-true
                          n286 = Equal?(x=w585, y=w582) -> (x = y?=w584:bool)
                        }
                        n287 = property class="PmEnumParam"(reference=w580) -> (reference out=w577:refnum<k24>, "Options"=w579:refnum<k24>)  [unwired: 1 in, 1 out]
                        n288 = invoke class="PmReadOnlyObservableCollection`" method="get_Item"(reference=w579, "index"=w578) -> ("get_Item"=w576:refnum<k24>)  [unwired: 2 in, 3 out]
                        n289 = property class="PmEnumItem"(reference=w576) -> ("Value"=w575:i32)  [unwired: 1 in, 2 out]
                        n290 = property class="PmEnumParam"(reference=w577, "Current"=w576) -> ()  [unwired: 1 in, 2 out]
                        n291 = property class="DigNum (strict)"(reference=w574, "Value"=w575) -> ()  [unwired: 1 in, 2 out]
                      }
                    }
                    n292 = local read "Exposure Time"() -> (w564:dbl)
                    n293 = In Range and Coerce(upper limit=w569, x=w564, lower limit=w568) -> (coerced(x)=w565:dbl)  [unwired: 1 out]
                    n294 = property class="CameraSettings"(reference=w556, "Exposure"=w565) -> ()  [unwired: 1 in, 2 out]
                    n295 = property class="PmNumericParam`1[[System.UInt64"(reference=w567, "Current"=w565) -> (reference out=w566:refnum<k24>)  [unwired: 1 in, 1 out]
                    n296 = property class="PmNumericParam`1[[System.UInt64"(reference=w566) -> ("Current"=w563:u64)  [unwired: 1 in, 2 out]
                    n297 = local write "Exposure Time"(w563) -> ()
                  }
                }
              }
            }
          }
          event "Get ROI": Value Change {
            n298 = event-data() -> ()  [unwired: 1 in, 6 out]
            n299 = case shown="True" "Get ROI" {
              tunnel: w602 -> [w604 w607]
              tunnel: [w604 w606] -> w601
              frame False {
              }
              frame True {
                n300 = local read "Camera Status"() -> (w605:bool)
                n301 = case shown="True" w605 {
                  tunnel: w607 -> [w609 w613]
                  tunnel: [w609 w610] -> w606
                  frame False {
                    n302 = One Button Dialog(message="Camera is not open") -> ()  [unwired: 1 in, 1 out]
                  }
                  frame True {
                    w618 = 0 items=["Idle", "Capturing"] ("Status")
                    n303 = property class="Camera"(reference=w613) -> (reference out=w612:refnum<k24>, "IsOpen"=w617:bool, "Status"=w619:i32)  [unwired: 1 in, 1 out]
                    n304 = Equal?(x=w617, y=TRUE) -> (x = y?=w615:bool)
                    n305 = Equal?(x=w619, y=w618) -> (x = y?=w614:bool)
                    n306 = Equal?(x=w615, y=w614) -> (x = y?=w611:bool)
                    n307 = case shown="True" w611 {
                      tunnel: w612 -> [w621 w629]
                      tunnel: [w621 w628] -> w610
                      frame False {
                        n308 = One Button Dialog(message="Camera must be idle.") -> ()  [unwired: 1 in, 1 out]
                      }
                      frame True {
                        n309 = property class="Camera"(reference=w629) -> (reference out=w628:refnum<k24>, "Settings"=w627:refnum<k24>)  [unwired: 1 in, 1 out]
                        n310 = property class="CameraSettings"(reference=w627) -> ("Regions"=w626:refnum<k24>)  [unwired: 1 in, 2 out]
                        n311 = property class="PmObservableCollection`1[[PVCam"(reference=w626) -> (reference out=w622:refnum<k24>, "Count"=w625:i32)  [unwired: 1 in, 1 out]
                        n312 = Greater?(x=w625, y=0) -> (0:w623:bool)
                        n313 = case shown="True" w623 {
                          tunnel: w622 -> [_ w631]
                          frame False {
                            n314 = One Button Dialog(message="ROI is not created.") -> ()  [unwired: 1 in, 1 out]
                          }
                          frame True {
                            n315 = invoke class="PmObservableCollection`1[[PVCam" method="get_Item"(reference=w631, "index"=0) -> ("get_Item"=w637:refnum<k24>)  [unwired: 2 in, 3 out]
                            n316 = property class="PmRegion"(reference=w637) -> ("Height"=w635:u16, "Width"=w634:u16, "X"=w633:u16, "Y"=w632:u16)  [unwired: 1 in, 2 out]
                            n317 = local write "Height"(w635) -> ()
                            n318 = local write "Width"(w634) -> ()
                            n319 = local write "X"(w633) -> ()
                            n320 = local write "Y"(w632) -> ()
                          }
                        }
                      }
                    }
                  }
                }
              }
            }
          }
          event "X", "Width", "Y", "Height": Value Change {
            n321 = event-data() -> ()  [unwired: 1 in, 6 out]
            n322 = local read "Camera Status"() -> (w640:bool)
            n323 = case shown="True" w640 {
              tunnel: w639 -> [w641 w644]
              tunnel: [w641 w642] -> w638
              frame False {
              }
              frame True {
                w650 = 0 items=["Idle", "Capturing"] ("Status")
                n324 = property class="Camera"(reference=w644) -> (reference out=w643:refnum<k24>, "IsOpen"=w649:bool, "Status"=w651:i32)  [unwired: 1 in, 1 out]
                n325 = Equal?(x=w649, y=TRUE) -> (x = y?=w647:bool)
                n326 = Equal?(x=w651, y=w650) -> (x = y?=w646:bool)
                n327 = Equal?(x=w647, y=w646) -> (x = y?=w645:bool)
                n328 = case shown="True" w645 {
                  tunnel: w643 -> [w652 w654]
                  tunnel: [w652 w653] -> w642
                  frame False {
                  }
                  frame True {
                    n329 = flat-sequence {
                      tunnel: w654 -> [w702]
                      tunnel: [w701] -> w653
                      frame #0 {
                        # "if (!( x >= 0\n            && (x+width) <= full_width\n            &&  0 < width \n            && y >= 0\n            && (y+height) <= full_height\n            && 0 < height ))\n        {\n           printf(\"Incorrect range for a ROI. \\n\");\n        }"
                        n330 = local read "Width"() -> (w670:u16)
                        n331 = local read "Height"() -> (w668:u16)
                        n332 = local read "Full CCD Height"() -> (w664:u16)
                        n333 = local read "Full CCD Width"() -> (w666:u16)
                        n334 = local read "X"() -> (w671:u16)
                        n335 = local read "Y"() -> (w667:u16)
                        n336 = local read "Height"() -> (w659:u16)
                        n337 = Add(x=w671, y=w670) -> (x+y=w665:u16)
                        n338 = local read "Width"() -> (w662:u16)
                        n339 = Add(x=w668, y=w667) -> (x+y=w663:u16)
                        n340 = local read "X"() -> (w672:u16)
                        n341 = local read "Y"() -> (w669:u16)
                        n342 = Less Or Equal?(x=w663, y=w664) -> (x <= y?=w679:bool)
                        n343 = Less Or Equal?(x=w665, y=w666) -> (x <= y?=w682:bool)
                        n344 = Less?(x=u16 0 ("y"), y=w659) -> (x < y?=w678:bool)
                        n345 = Greater Or Equal?(x=w672, y=u16 0) -> (x >= y?=w683:bool)
                        n346 = Less?(x=u16 0 ("y"), y=w662) -> (x < y?=w681:bool)
                        n347 = Greater Or Equal?(x=w669, y=u16 0) -> (x >= y?=w680:bool)
                        n348 = And(x=w679, y=w678) -> (x .and. y?=w674:bool)
                        n349 = And(x=w683, y=w682) -> (x .and. y?=w677:bool)
                        n350 = And(x=w681, y=w680) -> (x .and. y?=w676:bool)
                        n351 = And(x=w677, y=w676) -> (x .and. y?=w675:bool)
                        n352 = And(x=w675, y=w674) -> (x .and. y?=w673:bool)
                        n353 = case shown="False" w673 {
                          tunnel: [w687 w694] -> w658
                          tunnel: [u16 0 ("X") w693] -> w655
                          tunnel: [u16 0 ("Y") w692] -> w656
                          tunnel: [w688 w691] -> w657
                          frame False {
                            n354 = local read "Full CCD Height"() -> (w688:u16)
                            n355 = local read "Full CCD Width"() -> (w687:u16)
                            n356 = One Button Dialog(message="Wrong ROI ! Resetting to full CCD") -> ()  [unwired: 1 in, 1 out]
                          }
                          frame True {
                            n357 = local read "Height"() -> (w691:u16)
                            n358 = local read "Width"() -> (w694:u16)
                            n359 = local read "X"() -> (w693:u16)
                            n360 = local read "Y"() -> (w692:u16)
                          }
                        }
                        n361 = local write "Width"(w658) -> ()
                        n362 = local write "X"(w655) -> ()
                        n363 = local write "Y"(w656) -> ()
                        n364 = local write "Height"(w657) -> ()
                      }
                      frame #1 {
                        n365 = property class="Camera"(reference=w702) -> (reference out=w701:refnum<k24>, "Settings"=w700:refnum<k24>)  [unwired: 1 in, 1 out]
                        n366 = property class="CameraSettings"(reference=w700) -> ("Regions"=w699:refnum<k24>)  [unwired: 1 in, 2 out]
                        n367 = property class="PmObservableCollection`1[[PVCam"(reference=w699) -> (reference out=w695:refnum<k24>, "Count"=w698:i32)  [unwired: 1 in, 1 out]
                        n368 = Greater?(x=w698, y=0) -> (0:w696:bool)
                        n369 = case shown="True" w696 {
                          tunnel: w695 -> [_ w708]
                          frame False {
                            n370 = One Button Dialog(message="ROI is not created.") -> ()  [unwired: 1 in, 1 out]
                          }
                          frame True {
                            n371 = invoke class="PmObservableCollection`1[[PVCam" method="get_Item"(reference=w708, "index"=0) -> ("get_Item"=w710:refnum<k24>)  [unwired: 2 in, 3 out]
                            n372 = local read "Height"() -> (w707:u16)
                            n373 = local read "Width"() -> (w706:u16)
                            n374 = local read "X"() -> (w705:u16)
                            n375 = local read "Y"() -> (w704:u16)
                            n376 = property class="PmRegion"(reference=w710, "Height"=w707, "Width"=w706, "X"=w705, "Y"=w704) -> ()  [unwired: 1 in, 2 out]
                          }
                        }
                      }
                    }
                  }
                }
              }
            }
          }
          event "Path", "FramesToCapture": Value Change {
            n377 = event-data() -> ()  [unwired: 1 in, 6 out]
            n378 = local read "Camera Status"() -> (w713:bool)
            n379 = case shown="True" w713 {
              tunnel: w712 -> [w714 w717]
              tunnel: [w714 w715] -> w711
              frame False {
              }
              frame True {
                w723 = 0 items=["Idle", "Capturing"] ("Status")
                n380 = property class="Camera"(reference=w717) -> (reference out=w716:refnum<k24>, "IsOpen"=w722:bool, "Status"=w724:i32)  [unwired: 1 in, 1 out]
                n381 = Equal?(x=w722, y=TRUE) -> (x = y?=w720:bool)
                n382 = Equal?(x=w724, y=w723) -> (x = y?=w719:bool)
                n383 = Equal?(x=w720, y=w719) -> (x = y?=w718:bool)
                n384 = case shown="True" w718 {
                  tunnel: w716 -> [w725 w728]
                  tunnel: [w725 w727] -> w715
                  frame False {
                  }
                  frame True {
                    n385 = property class="Camera"(reference=w728) -> (reference out=w727:refnum<k24>, "Settings"=w731:refnum<k24>, "AcquisitionBuffer"=w732:refnum<k24>)  [unwired: 1 in, 1 out]
                    n386 = Path To String(path="Path") -> (string=w735:string)
                    n387 = Concatenate Strings(w735, "\\" ("string")) -> (w737:string)
                    "SavingPath" <- w737
                    n388 = property class="AcqBuffer"(reference=w732, "BufferSize"="FramesToCapture", "ImageSavingPath"=w737, "BigTiffRequired"=FALSE) -> (reference out=w733:refnum<k24>)  [unwired: 1 in, 1 out]
                    n389 = property class="CameraSettings"(reference=w731, "FramesToCapture"="FramesToCapture") -> ()  [unwired: 1 in, 2 out]
                    n390 = property class="AcqBuffer"(reference=w733) -> ("ImageSavingPath"=w734:string)  [unwired: 1 in, 2 out]
                    n391 = local write "SavingPath"(w734) -> ()
                  }
                }
              }
            }
          }
          event "Full CCD": Value Change {
            n392 = event-data() -> ()  [unwired: 1 in, 6 out]
            n393 = case shown="True" "Full CCD" {
              tunnel: w739 -> [w741 w744]
              tunnel: [w741 w743] -> w738
              frame False {
              }
              frame True {
                n394 = local read "Camera Status"() -> (w742:bool)
                n395 = case shown="True" w742 {
                  tunnel: w744 -> [w746 w750]
                  tunnel: [w746 w747] -> w743
                  frame False {
                    n396 = One Button Dialog(message="Camera is not open") -> ()  [unwired: 1 in, 1 out]
                  }
                  frame True {
                    w755 = 0 items=["Idle", "Capturing"] ("Status")
                    n397 = property class="Camera"(reference=w750) -> (reference out=w749:refnum<k24>, "IsOpen"=w754:bool, "Status"=w756:i32)  [unwired: 1 in, 1 out]
                    n398 = Equal?(x=w754, y=TRUE) -> (x = y?=w752:bool)
                    n399 = Equal?(x=w756, y=w755) -> (x = y?=w751:bool)
                    n400 = Equal?(x=w752, y=w751) -> (x = y?=w748:bool)
                    n401 = case shown="True" w748 {
                      tunnel: w749 -> [w757 w766]
                      tunnel: [w757 w765] -> w747
                      frame False {
                      }
                      frame True {
                        n402 = property class="Camera"(reference=w766) -> (reference out=w765:refnum<k24>, "Settings"=w764:refnum<k24>)  [unwired: 1 in, 1 out]
                        n403 = property class="CameraSettings"(reference=w764) -> (reference out=w758:refnum<k24>, "Regions"=w759:refnum<k24>)  [unwired: 1 in, 1 out]
                        n404 = property class="PmObservableCollection`1[[PVCam"(reference=w759) -> (reference out=w760:refnum<k24>, "Count"=w763:i32)  [unwired: 1 in, 1 out]
                        n405 = Greater?(x=w763, y=0) -> (0:w761:bool)
                        n406 = case shown="True" w761 {
                          tunnel: w760 -> [_ _]
                          tunnel: w759 -> [_ w775]
                          tunnel: w758 -> [_ w769]
                          frame False {
                          }
                          frame True {
                            n407 = invoke class="PmObservableCollection`1[[PVCam" method="RemoveAt"(reference=w775, "index"=0) -> ()  [unwired: 2 in, 4 out]
                            n408 = property class="CameraSettings"(reference=w769) -> ("SensorWidth"=w771:refnum<k24>)  [unwired: 1 in, 2 out]
                            n409 = property class="CameraSettings"(reference=w769) -> ("SensorHeight"=w772:refnum<k24>)  [unwired: 1 in, 2 out]
                            n410 = property class="PmNumericParam`1[[System.UInt32"(reference=w771) -> ("Current"=w770:u32)  [unwired: 1 in, 2 out]
                            n411 = property class="PmNumericParam`1[[System.UInt32"(reference=w772) -> ("Current"=w773:u32)  [unwired: 1 in, 2 out]
                            n412 = local write "Y"(0 ("index")) -> ()
                            n413 = local write "Width"(w770) -> ()
                            n414 = local write "Height"(w773) -> ()
                            n415 = local write "X"(0 ("index")) -> ()
                          }
                        }
                      }
                    }
                  }
                }
              }
            }
          }
          event "Live start": Value Change {
            n416 = event-data() -> ()  [unwired: 1 in, 6 out]
            n417 = case shown="True" "Live start" {
              tunnel: w778 -> [w780 w783]
              tunnel: [w780 w782] -> w777
              frame False {
              }
              frame True {
                n418 = local read "Camera Status"() -> (w781:bool)
                n419 = case shown="True" w781 {
                  tunnel: w783 -> [w784 w789]
                  tunnel: [w784 w787] -> w782
                  frame False {
                    n420 = One Button Dialog(message="Camera is not open") -> ()  [unwired: 1 in, 1 out]
                  }
                  frame True {
                    w794 = 0 items=["Idle", "Capturing"] ("Status")
                    n421 = property class="Camera"(reference=w789) -> (reference out=w788:refnum<k24>, "IsOpen"=w793:bool, "Status"=w795:i32)  [unwired: 1 in, 1 out]
                    n422 = Equal?(x=w793, y=TRUE) -> (x = y?=w791:bool)
                    n423 = Equal?(x=w795, y=w794) -> (x = y?=w790:bool)
                    n424 = Equal?(x=w791, y=w790) -> (x = y?=w786:bool)
                    n425 = case shown="True" w786 {
                      tunnel: w788 -> [w797 w799]
                      tunnel: [w797 w800] -> w787
                      frame False {
                        n426 = local write "Live"(FALSE ("Live 2")) -> ()
                      }
                      frame True {
                        n427 = flat-sequence {
                          tunnel: w799 -> [w805]
                          tunnel: [w802] -> w798
                          frame #0 {
                            n428 = property class="Camera"(reference=w805) -> (reference out=w802:refnum<k24>, "AcquisitionBuffer"=w804:refnum<k24>)  [unwired: 1 in, 1 out]
                            n429 = property class="AcqBuffer"(reference=w804, "BufferSize"=100) -> ()  [unwired: 1 in, 2 out]
                          }
                        }
                        n430 = local write "Live"(TRUE ("Live")) -> ()
                        n431 = invoke class="Camera" method="StartLive"(reference=w798) -> (reference out=w800:refnum<k24>)  [unwired: 2 in, 2 out]
                      }
                    }
                  }
                }
              }
            }
          }
          event "Live stop": Value Change {
            n432 = event-data() -> ()  [unwired: 1 in, 6 out]
            n433 = case shown="True" "Live stop" {
              tunnel: w807 -> [w809 w812]
              tunnel: [w809 w811] -> w806
              frame False {
              }
              frame True {
                n434 = local read "Camera Status"() -> (w810:bool)
                n435 = case shown="True" w810 {
                  tunnel: w812 -> [w814 w824]
                  tunnel: [w814 w821] -> w811
                  frame False {
                    n436 = One Button Dialog(message="Camera is not open") -> ()  [unwired: 1 in, 1 out]
                  }
                  frame True {
                    w819 = 1 items=["Idle", "Capturing"] ("Status")
                    n437 = property class="Camera"(reference=w824) -> (reference out=w822:refnum<k24>, "IsOpen"=w818:bool, "Status"=w820:i32)  [unwired: 1 in, 1 out]
                    n438 = Equal?(x=w820, y=w819) -> (x = y?=w815:bool)
                    n439 = Equal?(x=w818, y=TRUE) -> (x = y?=w816:bool)
                    n440 = Equal?(x=w816, y=w815) -> (x = y?=w823:bool)
                    n441 = case shown="True" w823 {
                      tunnel: w822 -> [w825 w828]
                      tunnel: [w825 w827] -> w821
                      frame False {
                      }
                      frame True {
                        n442 = invoke class="Camera" method="Stop"(reference=w828) -> (reference out=w827:refnum<k24>)  [unwired: 2 in, 2 out]
                        n443 = local write "Live"(FALSE ("Live 2")) -> ()
                      }
                    }
                  }
                }
              }
            }
          }
          event "Uninit": Value Change {
            n444 = event-data() -> ()  [unwired: 1 in, 6 out]
            n445 = case shown="True" "Uninit" {
              tunnel: w833 -> [w835 w839]
              tunnel: [w835 w838] -> w832
              tunnel: [FALSE ("Camera Status") w836] -> w830
              frame False {
              }
              frame True {
                n446 = local read "Camera Status"() -> (w837:bool)
                n447 = case shown="True" w837 {
                  tunnel: w839 -> [w841 w846]
                  tunnel: [w841 w845] -> w838
                  tunnel: [FALSE ("Camera Status") w844] -> w836
                  frame False {
                  }
                  frame True {
                    n448 = local read "Live"() -> (w842:bool)
                    n449 = Not(x=w842) -> (.not. x?=w843:bool)
                    n450 = case shown="True" w843 {
                      tunnel: w846 -> [w848 w851]
                      tunnel: [w848 w850] -> w845
                      tunnel: [FALSE ("Camera Status") w849] -> w844
                      frame False {
                      }
                      frame True {
                        n451 = flat-sequence {
                          tunnel: w851 -> [w854]
                          tunnel: [w853] -> w852
                          tunnel: [w857] -> w850
                          tunnel: w852 -> [w857]
                          tunnel: [TRUE ("Camera Status")] -> w849
                          frame #0 {
                            n452 = invoke class="Camera" method="Close"(reference=w854) -> (reference out=w853:refnum<k24>)  [unwired: 2 in, 2 out]
                          }
                          frame #1 {
                            n453 = local write "Camera Status"(FALSE ("Camera Status")) -> ()
                          }
                        }
                      }
                    }
                  }
                }
              }
            }
          }
        }
      }
    }
    frame #2 {
      n454 = invoke class="Library" method="Release"(reference=w859) -> (reference out=w860:refnum<k24>)  [unwired: 2 in, 2 out]
      n455 = Wait (ms)(milliseconds to wait=u32 100) -> ()  [unwired: 1 out]
      n456 = Close Reference(reference=w860) -> ()  [unwired: 1 in, 1 out]
    }
    frame #3 {
      n457 = invoke class="GC" method="Collect"() -> ()  [unwired: 3 in, 3 out]
    }
  }
  n458 = control-ref of="Exp. out"() -> (w7:refnum<vi>)
  n459 = property class="DigNum (strict)"(reference=w7, "Visible"=FALSE) -> ()  [unwired: 1 in, 2 out]
  n460 = control-ref of="Trigger Mode"() -> (w6:refnum<vi>)
  n461 = property class="DigNum (strict)"(reference=w6, "Visible"=FALSE) -> ()  [unwired: 1 in, 2 out]
  n462 = control-ref of="Trigger Out Behaviour"() -> (w12:refnum<vi>)
  n463 = control-ref of="Exp. out"() -> (w10:refnum<vi>)
  n464 = property class="DigNum (strict)"(reference=w10, "Value"=0) -> ()  [unwired: 1 in, 2 out]
  n465 = property class="CmbBox"(reference=w12, "Value"="") -> ()  [unwired: 1 in, 2 out]
  n466 = local write "Camera Status"(FALSE ("Camera Status")) -> ()
  n467 = property on="Scan Width" class="DigNum (strict)"("DisabledEnum"=w15) -> ()  [unwired: 2 in, 2 out]
  n468 = property on="Scan Line Delay" class="DigNum (strict)"("DisabledEnum"=w15) -> ()  [unwired: 2 in, 2 out]
  n469 = control-ref of="Scan Line Delay"() -> (w18:refnum<vi>)
  n470 = control-ref of="Scan Width"() -> (w21:refnum<vi>)
  n471 = control-ref of="Scan Line Time"() -> (w17:refnum<vi>)
  n472 = control-ref of="Scan Direction"() -> (w24:refnum<vi>)
  n473 = control-ref of="Scan Mode"() -> (w27:refnum<vi>)
  n474 = property class="CmbBox"(reference=w27, "Value"="", "Strings[]"=string[] [] ("Strings []")) -> ()  [unwired: 1 in, 2 out]
  n475 = property class="DigNum (strict)"(reference=w18, "Value"=0.0) -> ()  [unwired: 1 in, 2 out]
  n476 = property class="CmbBox"(reference=w24, "Strings[]"=string[] [] ("Strings []"), "Value"="") -> ()  [unwired: 1 in, 2 out]
  n477 = property class="DigNum (strict)"(reference=w21, "Value"=0.0) -> ()  [unwired: 1 in, 2 out]
  n478 = property class="DigNum (strict)"(reference=w17, "Value"=0.0) -> ()  [unwired: 1 in, 2 out]
  n479 = local write "Scan Direction Reset"(FALSE ("Boolean")) -> ()
  n480 = control-ref of="FramesToCapture"() -> (w4:refnum<vi>)
  n481 = property class="DigNum (strict)"(reference=w4, "Value"=10) -> ()  [unwired: 1 in, 2 out]
  "Boolean" <- FALSE ("Boolean")
  "Saving" <- FALSE ("Boolean")
  "Capturing" <- FALSE ("Boolean")
